vi "builder_options.vi"(8 "error in (no error)":errorcluster, 9 "path_index":i32, 10 "configuration":string, 11 "system.logging.provider in":refnum<class "system.logging.provider.lvclass">) -> (0 "error out":errorcluster, 3 "system.logging.provider out":refnum<class "system.logging.provider.lvclass">)   [LabVIEW 2021, in "system.logging.provider.lvclass"]
uses:
  system.logging.provider.lvclass
  system.logging.provider.lvclass/system.logging.provider.ctl
panel:
  # "Default behavior is no options loaded."
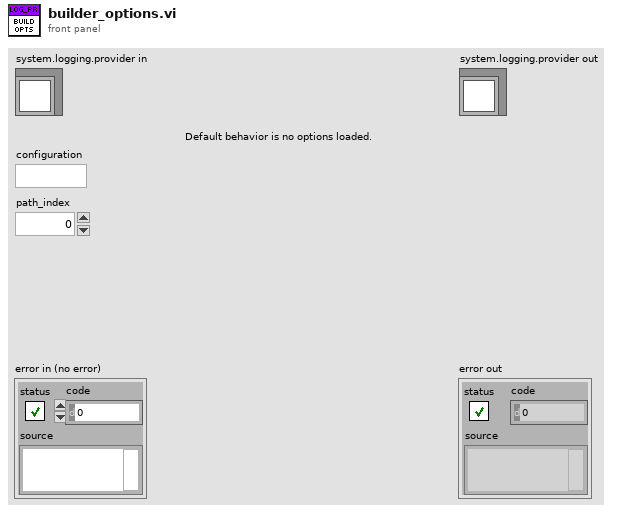
[diagram p1: front panel]
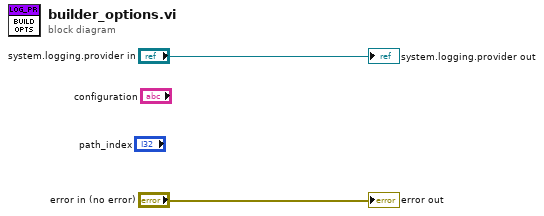
[diagram p0: block diagram]
diagram:
  "error out" <- "error in (no error)"
  "system.logging.provider out" <- "system.logging.provider in"
